vi "Configure Marker Type (Swept SA).vi"(0 "VISA resource name":refnum<visa-resource-name>, 1 "Manual Gate Time (0.1 s)":dbl=0.1, 2 "Auto Gate Time (T: Enable)":bool=TRUE, 5 "Active Marker (1: Marker1)":i32(ring)=1 items=["Marker1"=1, "Marker2"=2, "Marker3"=3, "Marker4"=4, "Marker5"=5, "Marker6"=6, "Marker7"=7, "Marker8"=8, "Marker9"=9, "Marker10"=10, "Marker11"=11, "Marker12"=12], 7 "Marker Type (0: Normal)":i32(ring) items=["Normal", "Delta", "Fixed", "Off"], 9 "Readout (0: Auto)":i32(ring) items=["Auto", "Frequency", "Period", "Time", "Inverse Time"], 11 "error in (no error)":errorcluster, 12 "Reference Marker (12: Marker12)":i32(ring)=12 items=["Marker1"=1, "Marker2"=2, "Marker3"=3, "Marker4"=4, "Marker5"=5, "Marker6"=6, "Marker7"=7, "Marker8"=8, "Marker9"=9, "Marker10"=10, "Marker11"=11, "Marker12"=12], 13 "Enable Marker Frequency Counter (F: Disable)":bool) -> (4 "VISA resource name out":refnum<visa-resource-name>, 15 "error out":errorcluster)   [LabVIEW 2018, in "Agilent MXA Series.lvlib"]
doc: "Configures the marker type on the spectrum analyzer.\n\n<B>Note:</B>\nYou can use this VI under the Swept SA mesasurement type on the spectrum analyzer."
uses:
  Agilent MXA Series.lvlib
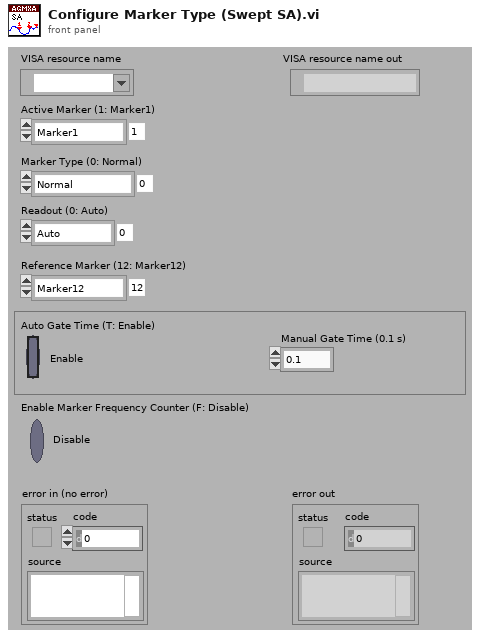
[diagram p1: front panel]
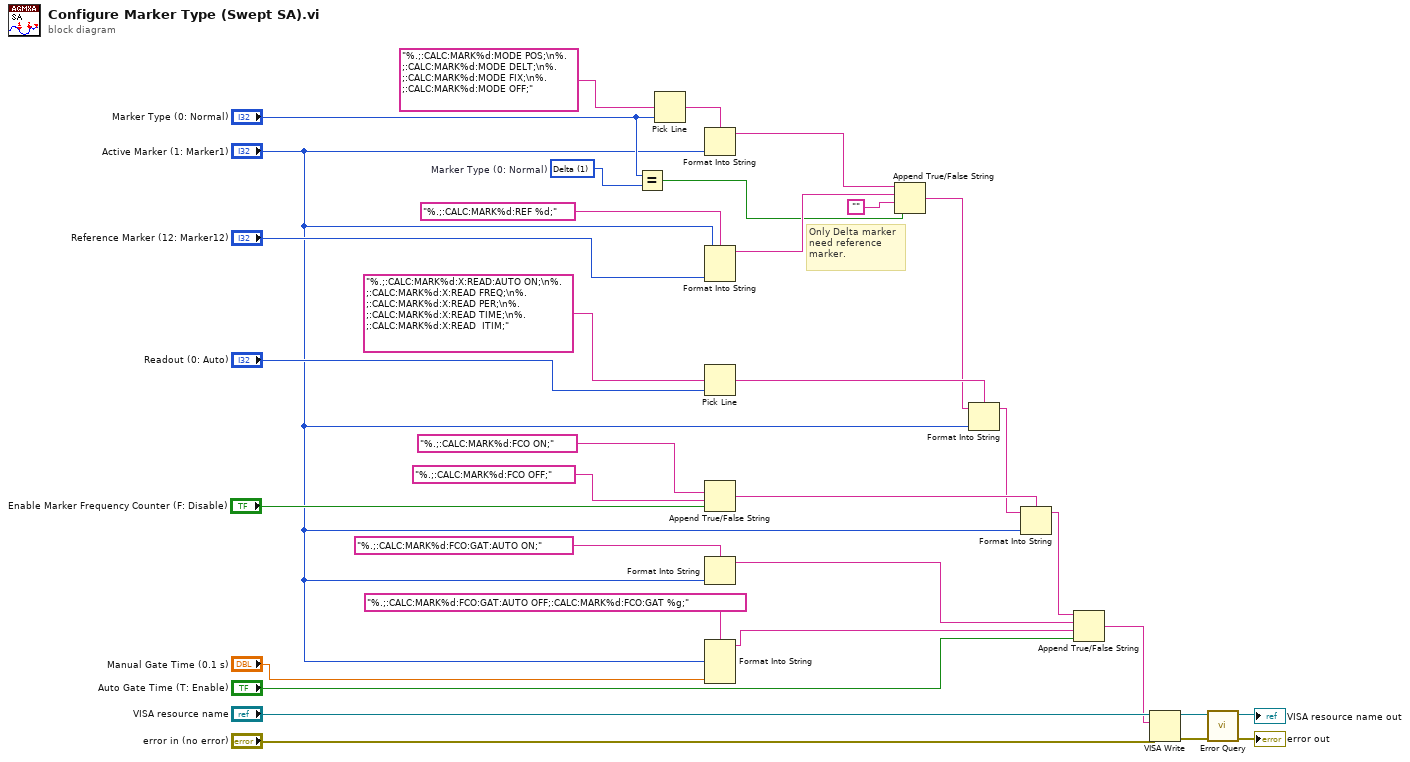
[diagram p0: block diagram]
diagram:
  w5 = 1 items=["Normal", "Delta", "Fixed", "Off"]  # Marker Type (0: Normal)
  # "Only Delta marker\nneed reference \nmarker."
  n1 = Equal?(x="Marker Type (0: Normal)", y=w5) -> (x = y?=w30:bool)
  n2 = Pick Line(multi-line string="%.;:CALC:MARK%d:MODE POS;\n%.;:CALC:MARK%d:MODE DELT;\n%.;:CALC:MARK%d:MODE FIX;\n%.;:CALC:MARK%d:MODE OFF;" ("Marker Type"), line index="Marker Type (0: Normal)") -> (output string=w33:string)  [unwired: 1 in]
  n3 = Format Into String(format string=w33, "Active Marker (1: Marker1)") -> (resulting string=w9:string)  [unwired: 2 in, 1 out]
  n4 = Format Into String(format string="%.;:CALC:MARK%d:REF %d;", "Active Marker (1: Marker1)", "Reference Marker (12: Marker12)") -> (resulting string=w31:string)  [unwired: 2 in, 1 out]
  n5 = Pick Line(multi-line string="%.;:CALC:MARK%d:X:READ:AUTO ON;\n%.;:CALC:MARK%d:X:READ FREQ;\n%.;:CALC:MARK%d:X:READ PER;\n%.;:CALC:MARK%d:X:READ TIME;\n%.;:CALC:MARK%d:X:READ  ITIM;" ("Marker Readout"), line index="Readout (0: Auto)") -> (output string=w25:string)  [unwired: 1 in]
  n6 = Append True/False String(1:"Enable Marker Frequency Counter (F: Disable)", 2:"%.;:CALC:MARK%d:FCO OFF;" ("false string"), 3:"%.;:CALC:MARK%d:FCO ON;" ("true string")) -> (0:w3:string)  [unwired: 1 in]
  n7 = Format Into String(format string="%.;:CALC:MARK%d:FCO:GAT:AUTO ON;", "Active Marker (1: Marker1)") -> (resulting string=w17:string)  [unwired: 2 in, 1 out]
  n8 = Format Into String(format string="%.;:CALC:MARK%d:FCO:GAT:AUTO OFF;:CALC:MARK%d:FCO:GAT %g;", "Active Marker (1: Marker1)", "Active Marker (1: Marker1)", "Manual Gate Time (0.1 s)") -> (resulting string=w16:string)  [unwired: 2 in, 1 out]
  n9 = Append True/False String(1:w30, 2:"", 3:w31, 4:w9) -> (0:w24:string)
  n10 = Format Into String(format string=w25, initial string=w24, "Active Marker (1: Marker1)") -> (resulting string=w2:string)  [unwired: 1 in, 1 out]
  n11 = Format Into String(format string=w3, initial string=w2, "Active Marker (1: Marker1)") -> (resulting string=w1:string)  [unwired: 1 in, 1 out]
  n12 = Append True/False String(1:"Auto Gate Time (T: Enable)", 2:w16, 3:w17, 4:w1) -> (0:w8:string)
  n13 = VISA Write(VISA resource name="VISA resource name", write buffer=w8, error in (no error)="error in (no error)") -> (VISA resource name out=w12:refnum<visa-resource-name>, error out=w13:errorcluster)  [unwired: 1 out]
  n14 = call "Error Query.vi"("error in (no error)"=w13, "VISA resource name"=w12) -> ("error out"=→"error out":errorcluster, "VISA resource name out"=→"VISA resource name out":refnum<visa-resource-name>)  [unwired: 6 in, 2 out]
